vi "RoutineResults.vi"() -> ()   [LabVIEW 2020]
doc: "This VI shows the results queried with the QueryFastRoutineResults.vi."
uses:
  C:/ProgramData/PI/LabVIEW/Low Level/GeneralCommands/Controller names.ctl
  Message Cluster.ctl
panel:
  out "Scan Results":T2(array[cluster]) {"Sys" min=1 step=1}
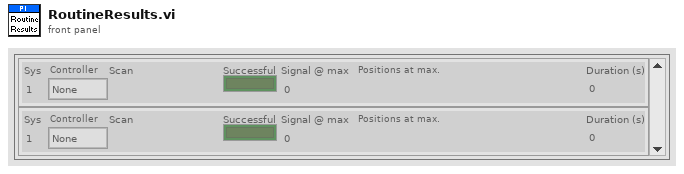
[diagram p1: front panel]
types:
  T1 = typedef "Controller names.ctl" = enum16{"None", "Analog", "C-702", "C-413", "C-414", "C-843", "C-843.PM", "C-844", "C-848", "C-865", "C-866", "C-867", "C-877", "C-880", "C-884", "C-885", "C-886", "C-887", "C-891", "E-135", "E-516", "E-517", "E-518", "E-709", "E-710", "E-712", "E-725", "E-727", "E-753", "E-754", "E-755", "E-761", "E-816", "E-861", "E-870", "E-871", "E-872", "E-873", "E-874", "F-206", "HydraPollux", "M-840", "M-850", "M-8X0", "Mercury", "Mercury_GCS", "PI_GCS2"}
  T2 = cluster{"Sys":i32, "Controller":T1, "Scan":string, "Successful":bool, "Signal @ max":dbl, "Positions at max.":string, "Duration (s)":dbl}[]
  T3 = typedef "Message Cluster.ctl" = cluster{"Message":string, "Message Data":variant}
  T4 = cluster{"Sys":i32, "Controller":T1, "Scan":string, "Successful":bool, "Signal Intensity at max":dbl, "Positions at max.":string, "Duration (s)":dbl}[]
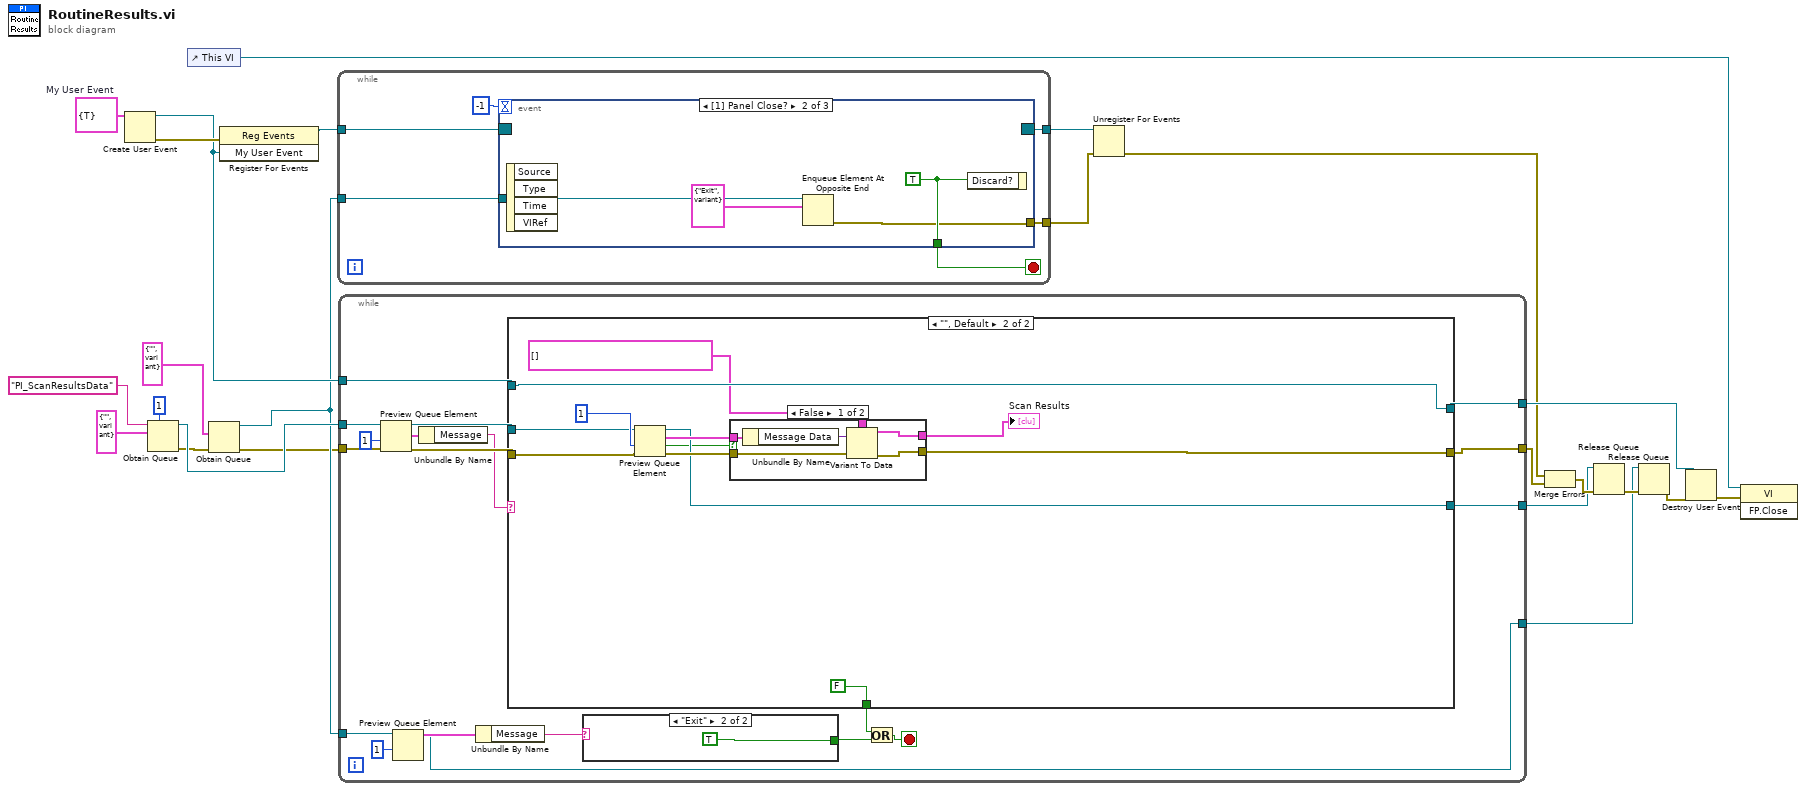
[diagram p0: block diagram]
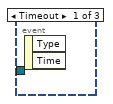
[diagram p2: hidden frame]
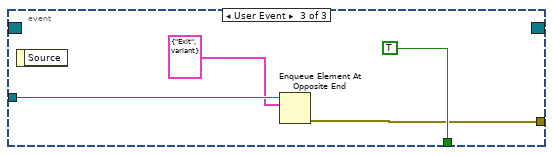
[diagram p3: hidden frame]
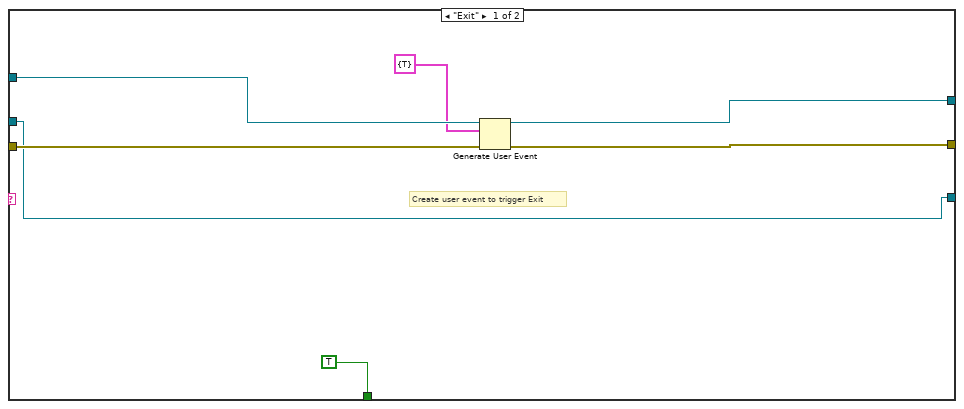
[diagram p4: hidden frame]
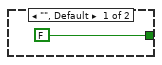
[diagram p6: hidden frame]
diagram:
  w6 = cluster{"Trigger":bool} {"Trigger"=TRUE}  # My User Event
  n1 = Create User Event(user event datatype=w6) -> (user event=w12:refnum<user-event>, error out=w13:errorcluster)  [unwired: 1 in]
  n2 = Obtain Queue(max queue size (-1, unlimited)=1, name (unnamed)="PI_ScanResultsData", element data type=T3 {"Message"="", "Message Data"=variant} ("Message Cluster")) -> (queue out=w18:refnum<queue>, error out=w5:errorcluster)  [unwired: 2 in, 1 out]
  n3 = control-ref of="This VI"() -> (w15:refnum<vi>)
  n4 = Obtain Queue(element data type=T3 {"Message"="", "Message Data"=variant} ("Message Cluster"), error in (no error)=w5) -> (queue out=w4:refnum<queue>, error out=w3:errorcluster)  [unwired: 2 in, 2 out]
  n5 = register-events(error in=w13, w12) -> (reference out=w14:refnum<event-registration>)  [unwired: 1 in, 1 out]
  n6 = while {
    tunnel: w4 -> [w29]
    tunnel: [w28] -> w10
    tunnel: w14 -> [w26]
    tunnel: [w25] -> w11
    stop <- w30 stop-if-true
    n7 = event shown="[1] Panel Close?" {
      selector: w26 -> [_ _ _]
      dyn-events: [_ _ _] -> w25
      timeout: -1 -> [_ _ _]
      tunnel: [_ w34 TRUE] -> w30
      tunnel: w29 -> [_ w33 w37]
      tunnel: [_ w31 w36] -> w28
      event Timeout {
        n8 = event-data() -> ()  [unwired: 3 out]
      }
      event Panel Close? {
        w34 = TRUE
        n9 = event-data() -> ()  [unwired: 5 out]
        n10 = Enqueue Element At Opposite End(queue=w33, element=T3 {"Message"="Exit", "Message Data"=variant}) -> (error out=w31:errorcluster)  [unwired: 1 in, 3 out]
        n11 = event-data("Discard?"=w34) -> ()  [unwired: 1 in, 1 out]
      }
      event User Event {
        n12 = event-data() -> ()  [unwired: 2 out]
        n13 = Enqueue Element At Opposite End(queue=w37, element=T3 {"Message"="Exit", "Message Data"=variant}) -> (error out=w36:errorcluster)  [unwired: 1 in, 3 out]
      }
    }
  }
  n14 = while {
    tunnel: w4 -> [w48]
    tunnel: w18 -> [w54]
    tunnel: [w40] -> w19
    tunnel: w12 -> [w43]
    tunnel: [w42] -> w7
    tunnel: [w41] -> w2
    tunnel: w3 -> [w52]
    tunnel: [w39] -> w24
    stop <- w44 stop-if-true
    n15 = Preview Queue Element(queue=w54, timeout in ms (-1)=1, error in (no error)=w52) -> (queue out=w53:refnum<queue>, element=w50:T3, error out=w51:errorcluster)  [unwired: 1 out]
    n16 = Preview Queue Element(queue=w48, timeout in ms (-1)=1) -> (queue out=w40:refnum<queue>, element=w57:T3)  [unwired: 1 in, 2 out]
    n17 = Unbundle By Name(w50) -> ("Message"=w49:string)
    n18 = Unbundle By Name(w57) -> ("Message"=w56:string)
    n19 = case shown="\"\", Default" w49 {
      tunnel: [w60 w70] -> w39
      tunnel: w53 -> [w58 w69]
      tunnel: w51 -> [w61 w71]
      tunnel: [TRUE FALSE] -> w45
      tunnel: w43 -> [w63 w75]
      tunnel: [w62 w75] -> w42
      tunnel: [w58 w66] -> w41
      frame "Exit" {
        # "Create user event to trigger Exit"
        n20 = Generate User Event(user event=w63, event data cluster=cluster{bool} {TRUE} ("event data"), error in=w61) -> (user event out=w62:refnum<user-event>, error out=w60:errorcluster)  [unwired: 1 in]
      }
      frame "", Default {
        n21 = Preview Queue Element(queue=w69, timeout in ms (-1)=1, error in (no error)=w71) -> (queue out=w66:refnum<queue>, element=w74:T3, timed out?=w65:bool, error out=w73:errorcluster)
        n22 = case shown="False" w65 {
          tunnel: w74 -> [w82 _]
          tunnel: w73 -> [w80 w84]
          tunnel: [w79 w84] -> w70
          tunnel: T4 [] ("Scan Results") -> [w78 w83]
          tunnel: [w77 w83] -> w67
          frame False {
            n23 = Unbundle By Name(w82) -> ("Message Data"=w81:variant)
            n24 = Variant To Data(error in=w80, type=w78, Variant=w81) -> (data=w77:T4, error out=w79:errorcluster)
          }
          frame True {
          }
        }
        "Scan Results" <- w67
      }
    }
    n25 = case shown="\"Exit\"" w56 {
      tunnel: [FALSE TRUE] -> w46
      frame "", Default {
      }
      frame "Exit" {
      }
    }
    n26 = Or(x=w45, y=w46) -> (x .or. y?=w44:bool)
  }
  n27 = Unregister For Events(event registration refnum=w11, error in=w10) -> (error out=w1:errorcluster)
  n28 = Merge Errors(w1, w24) -> (w23:errorcluster)
  n29 = Release Queue(queue=w2, error in (no error)=w23) -> (error out=w20:errorcluster)  [unwired: 3 out]
  n30 = Release Queue(queue=w19, error in (no error)=w20) -> (error out=w9:errorcluster)  [unwired: 3 out]
  n31 = Destroy User Event(user event=w7, error in=w9) -> (error out=w8:errorcluster)
  n32 = invoke class="VI" method="FP.Close"(reference=w15, error in=w8) -> ()  [unwired: 1 in, 3 out]
